vi "testSendEvtServersAandB.vi"(8 "error in (no error)":errorcluster) -> (0 "error out":errorcluster)   [LabVIEW 2018]
uses:
  src/FactoryTcpServer/FactoryTcpServer.lvclass
  src/TcpServer/TcpServer.lvclass/TcpServer.ctl
  src/TcpServerCmd/TcpServerCmd.lvclass/TcpServerCmd.ctl
  <vilib>/addons/_JKI Toolkits/Caraya/classes/Assert/Assert Equal Value_Variant.vi
  src/TcpServerCmd/TcpServerCmd.lvclass
  <vilib>/addons/_JKI Toolkits/Caraya/classes/Test/Test.lvclass
  <vilib>/addons/_JKI Toolkits/Caraya/classes/Assert/Assert.lvclass
  src/TcpServer/TcpServer.lvclass
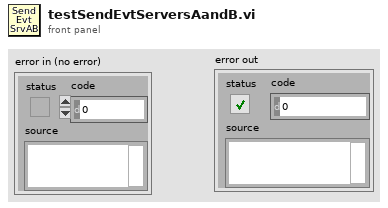
[diagram p1: front panel]
types:
  T1 = typedef "TcpServerCmd.lvclass/userEventTypeDef.ctl" = cluster{"CmdRead":refnum<user-event>, "CmdWrite":refnum<user-event>, "EvtRead":refnum<user-event>, "EvtWrite":refnum<user-event>}
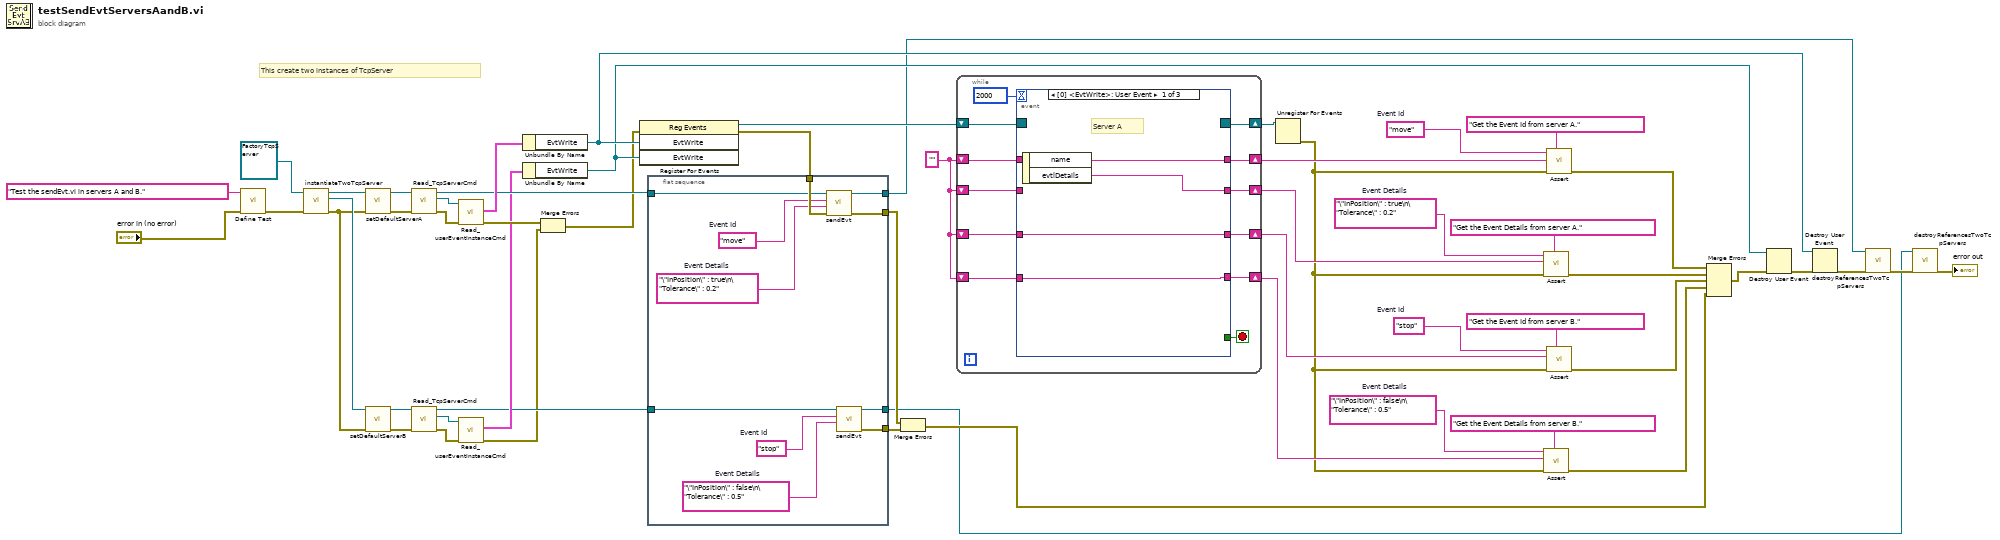
[diagram p0: block diagram]
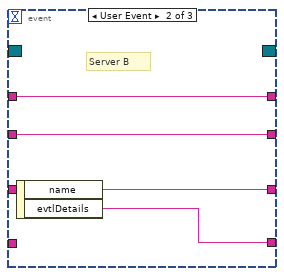
[diagram p2: hidden frame]
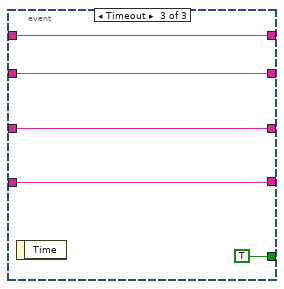
[diagram p3: hidden frame]
diagram:
  w18 = "" ("name")
  w27 = "\"InPosition\" : false\n\"Tolerance\" : 0.5"  # Event Details
  w26 = "stop"  # Event Id
  w42 = "\"InPosition\" : true\n\"Tolerance\" : 0.2"  # Event Details
  w43 = "move"  # Event Id
  # "This create two instances of TcpServer"
  n1 = call <vilib>:"Define Test.vi"("error in (no error)"="error in (no error)", "Label (VI Title)"="Test the sendEvt.vi in servers A and B.") -> ("error out"=w8:errorcluster)  [unwired: 9 in]
  n2 = call "instantiateTwoTcpServer.vi"("error in (no error)"=w8, "FactoryTcpServer in"=refnum<class "FactoryTcpServer.lvclass"> refnum) -> ("error out"=w5:errorcluster, "TcpServer 2 out"=w6:refnum<class "TcpServer.lvclass">, "TcpServer 1 out"=w7:refnum<class "TcpServer.lvclass">)  [unwired: 6 in, 1 out]
  n3 = call "setDefaultServerA.vi"("error in (no error)"=w5, "TcpServer.lvclass"=w7) -> ("error out"=w35:errorcluster, "tcpServer out"=w34:refnum<class "TcpServer.lvclass">)  [unwired: 8 in]
  n4 = call "setDefaultServerB.vi"("error in (no error)"=w5, "TcpServer.lvclass"=w6) -> ("error out"=w30:errorcluster, "tcpServer out"=w31:refnum<class "TcpServer.lvclass">)  [unwired: 8 in]
  n5 = call "Read_TcpServerCmd.vi"("error in (no error)"=w35, "TcpServer in"=w34) -> ("error out"=w40:errorcluster, "TcpServerCmd.lvclass"=w41:refnum<class "TcpServerCmd.lvclass">, "TcpServer out"=w36:refnum<class "TcpServer.lvclass">)  [unwired: 7 in]
  n6 = call "Read_TcpServerCmd.vi"("error in (no error)"=w30, "TcpServer in"=w31) -> ("error out"=w33:errorcluster, "TcpServerCmd.lvclass"=w32:refnum<class "TcpServerCmd.lvclass">, "TcpServer out"=w28:refnum<class "TcpServer.lvclass">)  [unwired: 7 in]
  n7 = call "Read_userEventInstanceCmd.vi"("error in (no error)"=w40, "TcpServerCmd in"=w41) -> ("error out"=w37:errorcluster, "userEventInstance"=w39:T1)  [unwired: 7 in, 1 out]
  n8 = call "Read_userEventInstanceCmd.vi"("error in (no error)"=w33, "TcpServerCmd in"=w32) -> ("error out"=w12:errorcluster, "userEventInstance"=w29:T1)  [unwired: 7 in, 1 out]
  n9 = Unbundle By Name(w39) -> ("EvtWrite"=w38:refnum<user-event>)
  n10 = Unbundle By Name(w29) -> ("EvtWrite"=w14:refnum<user-event>)
  n11 = Merge Errors(w37, w12) -> (w13:errorcluster)
  n12 = register-events(error in=w13, w38, w14) -> (reference out=w53:refnum<event-registration>, error out=w52:errorcluster)  [unwired: 1 in]
  n13 = flat-sequence {
    tunnel: w52 -> [w66]
    tunnel: w36 -> [w63]
    tunnel: w28 -> [w62]
    tunnel: [w59] -> w17
    tunnel: [w58] -> w10
    tunnel: [w57] -> w2
    tunnel: [w56] -> w1
    frame #0 {
      w60 = "\"InPosition\" : false\n\"Tolerance\" : 0.5"  # Event Details
      w61 = "stop"  # Event Id
      w64 = "\"InPosition\" : true\n\"Tolerance\" : 0.2"  # Event Details
      w65 = "move"  # Event Id
      n14 = call "sendEvt.vi"("error in (no error)"=w66, "Event Details"=w64, "Event Id"=w65, "tcpServer in"=w63) -> ("error out"=w58:errorcluster, "tcpServer out"=w57:refnum<class "TcpServer.lvclass">)  [unwired: 6 in]
      n15 = call "sendEvt.vi"("Event Details"=w60, "Event Id"=w61, "tcpServer in"=w62) -> ("error out"=w59:errorcluster, "tcpServer out"=w56:refnum<class "TcpServer.lvclass">)  [unwired: 7 in]
    }
  }
  n16 = Merge Errors(w10, w17) -> (w11:errorcluster)
  n17 = while {
    shift-right: [w75] -> w45
    shift-left: w53 -> [w78]
    shift-right: [w76] -> w48
    shift-left: w18 -> [w70]
    shift-right: [w77] -> w50
    shift-left: w18 -> [w69]
    shift-right: [w72] -> w23
    shift-left: w18 -> [w68]
    shift-right: [w71] -> w22
    shift-left: w18 -> [w67]
    stop <- w73 stop-if-true
    n18 = event shown="[0] <EvtWrite>: User Event" {
      selector: w78 -> [_ _ _]
      dyn-events: [_ _ _] -> w75
      timeout: 2000 -> [_ _ _]
      tunnel: [w82 w83 w89] -> w77
      tunnel: [w81 w84 w90] -> w76
      tunnel: [_ _ TRUE] -> w73
      tunnel: [w80 w86 w88] -> w72
      tunnel: [w79 w85 w87] -> w71
      tunnel: w70 -> [_ w84 w90]
      tunnel: w69 -> [_ w83 w89]
      tunnel: w68 -> [w80 _ w88]
      tunnel: w67 -> [w79 _ w87]
      event User Event {
        # "Server A"
        n19 = event-data() -> ("name"=w81:string, "evtlDetails"=w82:string)  [unwired: 1 in]
      }
      event User Event {
        # "Server B"
        n20 = event-data() -> ("name"=w86:string, "evtlDetails"=w85:string)  [unwired: 1 in]
      }
      event Timeout {
        n21 = event-data() -> ()  [unwired: 1 in, 1 out]
      }
    }
  }
  n22 = Unregister For Events(event registration refnum=w45) -> (error out=w21:errorcluster)  [unwired: 1 in]
  n23 = call-poly <vilib>:"Assert.vi"("Label"="Get the Event Details from server A.", "error in (no error)"=w21, "Y"=w50, "X"=w42) -> ("error out"=w47:errorcluster)  [unwired: 7 in]
  n24 = call-poly <vilib>:"Assert.vi"("Label"="Get the Event Details from server B.", "error in (no error)"=w21, "Y"=w22, "X"=w27) -> ("error out"=w19:errorcluster)  [unwired: 7 in]
  n25 = call-poly <vilib>:"Assert.vi"("Label"="Get the Event Id from server A.", "error in (no error)"=w21, "Y"=w48, "X"=w43) -> ("error out"=w46:errorcluster)  [unwired: 7 in]
  n26 = call-poly <vilib>:"Assert.vi"("Label"="Get the Event Id from server B.", "error in (no error)"=w21, "Y"=w23, "X"=w26) -> ("error out"=w20:errorcluster)  [unwired: 7 in]
  n27 = Merge Errors(w46, w47, w20, w19, w11) -> (w16:errorcluster)
  n28 = Destroy User Event(user event=w14, error in=w16) -> (error out=w15:errorcluster)
  n29 = Destroy User Event(user event=w38, error in=w15) -> (error out=w44:errorcluster)
  n30 = call "destroyReferencesTwoTcpServers.vi"("error in (no error)"=w44, "TcpServer in"=w2) -> ("error out"=w4:errorcluster)  [unwired: 8 in, 1 out]
  n31 = call "destroyReferencesTwoTcpServers.vi"("error in (no error)"=w4, "TcpServer in"=w1) -> ("error out"=→"error out":errorcluster)  [unwired: 8 in, 1 out]
